vi "Fiducial Scan.vi"(8 "error in":errorcluster, 10 "input cluster":T1, 11 "Gantry In":refnum<k24>) -> (0 "error out":errorcluster, 1 "Not Found?":bool, 2 "output cluster":T1, 3 "Gantry Out":refnum<k24>)   [LabVIEW 2021, in "Component Tray.lvclass"]
uses:
  Component Tray.lvclass
  Find Component.ctl
  Controller/Camera/Machine Vision.ctl
  C:/Program Files (x86)/Aerotech/A3200/LabVIEW/2010/Bin/Aerotech.A3200.dll
  Program Files (x86)/Aerotech/A3200/LabVIEW/2010/Bin/Aerotech.A3200.dll
  Controller/Motion/A3200/A3200.lvclass
  Controller/Camera/Camera.lvclass
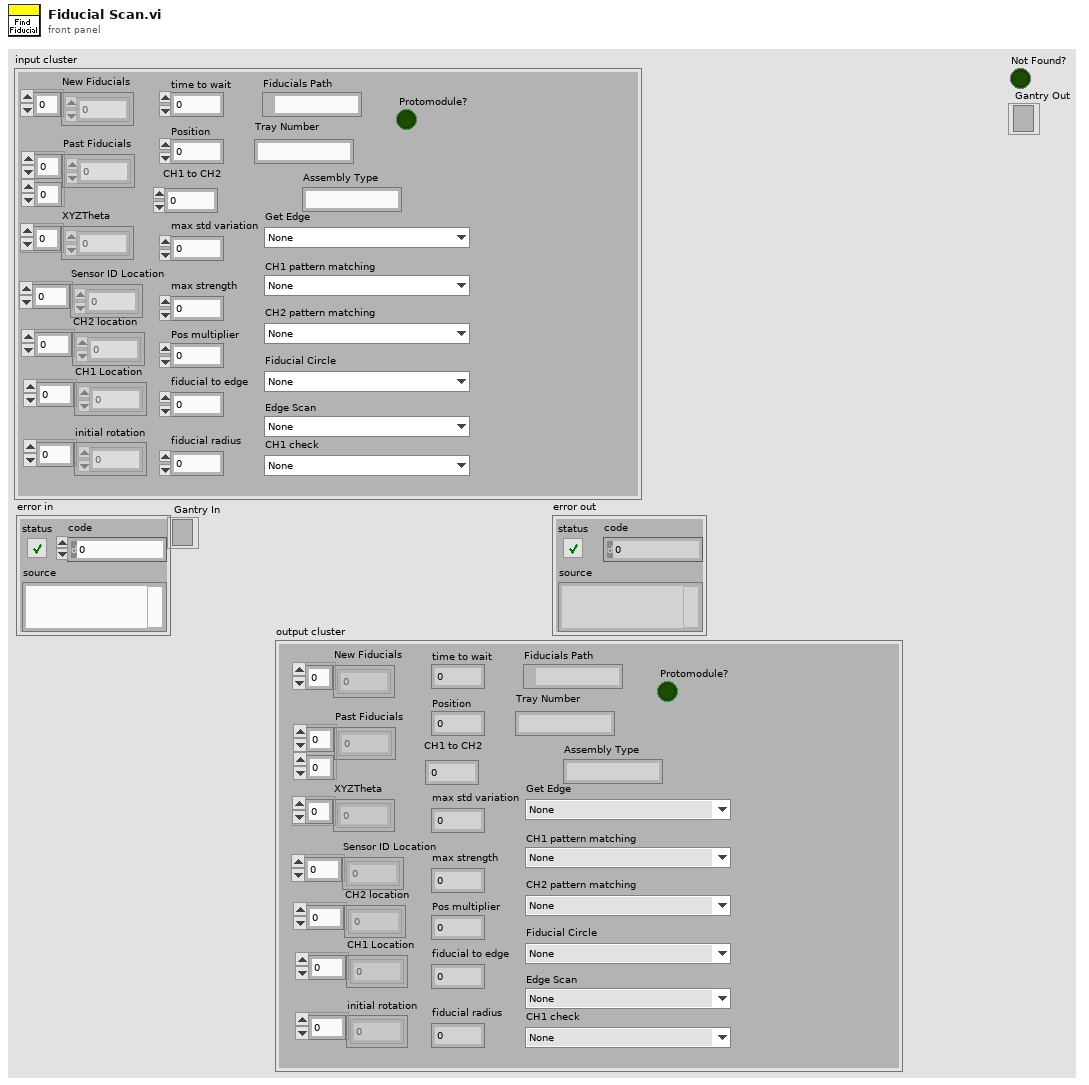
[diagram p1: front panel]
types:
  T1 = typedef "Component Tray.lvclass/Find Component.ctl" = cluster{"New Fiducials":dbl[], "Past Fiducials":dbl[][], "XYZTheta":dbl[], "Fiducials Path":path, "Position":i32, "CH1 Location":dbl[], "Sensor ID Location":dbl[], "initial rotation":dbl[], "CH2 location":dbl[], "max std variation":dbl, "max strength":dbl, "CH2 pattern matching":T2, "Fiducial Circle":T2, "Get Edge":T2, "Pos multiplier":dbl, "time to wait":u32, "fiducial to edge":dbl, "Protomodule?":bool, "Assembly Type":string, "CH1 to CH2":dbl, "Tray Number":string, "fiducial radius":dbl, "4 fiducials?":bool, "CH1 check":T2, "Edge Scan":T2, "CH1 pattern matching":T2, "Sensor Thickness":dbl}
  T2 = typedef "Camera.lvclass/Machine Vision.ctl" = enum16{"None", "Assembly Tray Circle", "Assembly Tray Fiducial", "Partial Hexaboard", "sensor edge init", "HB edge init", "sensor edge pos1", "sensor edge pos2", "HB edge pos1", "HB edge pos2", "Sensor CH1-2", "HB CH1", "HB CH2", "V3 Sensor Circle", "Hexaboard Circle", "sensor CH1 check", "HB CH1 check "}
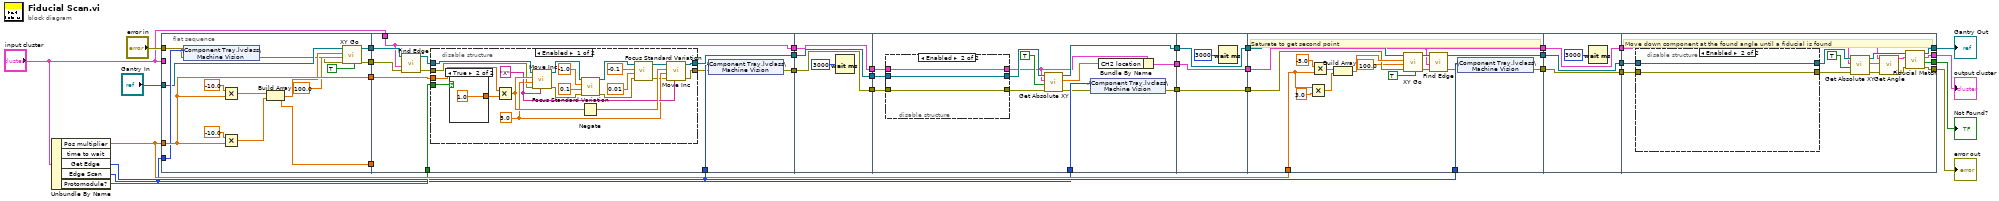
[diagram p0: block diagram]
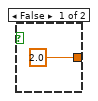
[diagram p2: hidden frame]
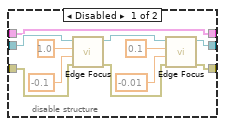
[diagram p4: hidden frame]
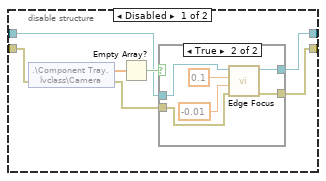
[diagram p5: hidden frame]
diagram:
  n1 = Unbundle By Name("input cluster") -> ("Pos multiplier"=w33:dbl, "Get Edge"=w2:T2, "Edge Scan"=w1:T2, "Protomodule?"=w6:bool)  [unwired: 1 out]
  n2 = flat-sequence {
    tunnel: w1 -> [w46]
    tunnel: w33 -> [w47]
    tunnel: "Gantry In" -> [w45]
    tunnel: [w34] -> w15
    tunnel: [w47] -> w14
    tunnel: [w35] -> w13
    tunnel: "error in" -> [w37]
    tunnel: [w38] -> w11
    tunnel: "input cluster" -> [_]
    tunnel: [w58] -> w5
    tunnel: [w55] -> w4
    tunnel: [w49] -> w3
    tunnel: w2 -> [w57]
    tunnel: w15 -> [w50]
    tunnel: w14 -> [w51]
    tunnel: w13 -> [w52]
    tunnel: w11 -> [_]
    tunnel: "input cluster" -> [w49]
    tunnel: w6 -> [w48]
    tunnel: w5 -> [w87]
    tunnel: [w87] -> w9
    tunnel: w4 -> [w86]
    tunnel: [w86] -> w8
    tunnel: [w84] -> w7
    tunnel: w3 -> [w84]
    tunnel: [w100] -> w21
    tunnel: [w96] -> w19
    tunnel: [w99] -> w17
    tunnel: w1 -> [w98]
    tunnel: w9 -> [w92]
    tunnel: w8 -> [w91]
    tunnel: w7 -> [w90]
    tunnel: w21 -> [w118]
    tunnel: [w118] -> w20
    tunnel: w19 -> [w117]
    tunnel: [w117] -> w18
    tunnel: w17 -> [w116]
    tunnel: [w116] -> w16
    tunnel: [w132] -> w27
    tunnel: [w135] -> w25
    tunnel: w2 -> [w134]
    tunnel: [w119] -> w23
    tunnel: w16 -> [w119]
    tunnel: w33 -> [w121]
    tunnel: w18 -> [w125]
    tunnel: w20 -> [w123]
    tunnel: w27 -> [w139]
    tunnel: [w139] -> w26
    tunnel: w25 -> [w138]
    tunnel: [w138] -> w24
    tunnel: w23 -> [w137]
    tunnel: [w137] -> w22
    tunnel: [w153] -> w32
    tunnel: [w152] -> w31
    tunnel: [w149] -> w29
    tunnel: [w148] -> w28
    tunnel: w22 -> [w141]
    tunnel: w24 -> [w145]
    tunnel: w26 -> [w143]
    frame #0 {
      n3 = shared-variable ".\\Component Tray.lvclass\\Machine Vision"(w46, error in=w37) -> (error out=w36:errorcluster)
      n4 = Multiply(x=-10.0, y=w47) -> (x*y=w42:dbl)
      n5 = Multiply(x=-10.0, y=w47) -> (x*y=w43:dbl)
      n6 = Build Array(w42, w43) -> (w38:dbl[])
      n7 = call "XY Go.vi"("Increment?"=TRUE, "error in (no error)"=w36, "Speed"=100.0, "XY In"=w38, "Gantry In"=w45) -> ("error out"=w34:errorcluster, "Gantry Out"=w35:refnum<k24>)  [unwired: 4 in, 1 out]
    }
    frame #1 {
      n8 = call "Find Edge.vi"("error in"=w50, "input cluster"=w49, "Gantry In"=w52) -> ("error out"=w53:errorcluster, "Gantry Out"=w54:refnum<k24>)  [unwired: 7 in]
      n9 = disable-structure shown="Enabled" {
        disable-tunnel: w54 -> [w77 w83]
        disable-tunnel: [w74 w83] -> w58
        disable-tunnel: [w69 w82] -> w56
        disable-tunnel: w53 -> [w60 w82]
        disable-tunnel: w51 -> [w79 _]
        disable-tunnel: w48 -> [w59 _]
        frame Enabled {
          w71 = "X" ("Axis")
          w70 = 5.0 ("Speed")
          n10 = case shown="True" w59 {
            tunnel: [2.0 ("y") 1.0 ("y")] -> w78
            frame False {
            }
            frame True {
            }
          }
          n11 = Multiply(x=w79, y=w78) -> (x*y=w73:dbl)
          n12 = call "Move Inc.vi"("Axis"=w71, "error in (no error)"=w60, "Speed"=w70, "Distance"=w73, "Gantry In"=w77) -> ("error out"=w75:errorcluster, "Gantry Out"=w76:refnum<k24>)  [unwired: 5 in]
          n13 = Negate(x=w73) -> (-x=w72:dbl)
          n14 = call "Focus Standard Variation.vi"("error in"=w75, "Scan Inc"=0.1, "Start Inc"=-1.0, "Gantry In"=w76) -> ("error out"=w68:errorcluster, "Gantry Out"=w66:refnum<k24>)  [unwired: 5 in, 1 out]
          n15 = call "Focus Standard Variation.vi"("error in"=w68, "Scan Inc"=0.01, "Start Inc"=-0.1, "Gantry In"=w66) -> ("error out"=w67:errorcluster, "Gantry Out"=w65:refnum<k24>)  [unwired: 5 in, 1 out]
          n16 = call "Move Inc.vi"("Axis"=w71, "error in (no error)"=w67, "Speed"=w70, "Distance"=w72, "Gantry In"=w65) -> ("error out"=w69:errorcluster, "Gantry Out"=w74:refnum<k24>)  [unwired: 5 in]
        }
        frame Disabled {
        }
      }
      n17 = shared-variable ".\\Component Tray.lvclass\\Machine Vision"(w57, error in=w56) -> (error out=w55:errorcluster)
    }
    frame #2 {
      n18 = Wait (ms)(milliseconds to wait=u32 3000) -> ()  [unwired: 1 out]
    }
    frame #3 {
      n19 = disable-structure shown="Enabled" {
        disable-tunnel: w92 -> [w111 w114]
        disable-tunnel: [w105 w114] -> w93
        disable-tunnel: [w104 w113] -> w94
        disable-tunnel: w91 -> [w110 w113]
        disable-tunnel: w90 -> [w109 w112]
        disable-tunnel: [w109 w112] -> w88
        frame Disabled {
          n20 = call "Edge Focus.vi"("error in"=w110, "Increment Size"=-0.1, "Position In"=1.0, "Gantry In"=w111) -> ("error out"=w103:errorcluster, "Gantry Out"=w106:refnum<k24>)  [unwired: 6 in]
          n21 = call "Edge Focus.vi"("error in"=w103, "Increment Size"=-0.01, "Position In"=0.1, "Gantry In"=w106) -> ("error out"=w104:errorcluster, "Gantry Out"=w105:refnum<k24>)  [unwired: 6 in]
        }
        frame Enabled {
        }
      }
      n22 = call "Get Absolute XY.vi"("error in (no error)"=w94, "Edge?"=TRUE, "input cluster"=w88, "Gantry In"=w93) -> ("error out"=w97:errorcluster, "Abs XY"=w95:dbl[], "Gantry Out"=w100:refnum<k24>)  [unwired: 5 in]
      n23 = shared-variable ".\\Component Tray.lvclass\\Machine Vision"(w98, error in=w97) -> (error out=w96:errorcluster)
      n24 = Bundle By Name(cluster=w88, "CH2 location"=w95) -> (w99:T1)
    }
    frame #4 {
      n25 = Wait (ms)(milliseconds to wait=u32 3000) -> ()  [unwired: 1 out]
    }
    frame #5 {
      # "Saturate to get second point"
      n26 = Multiply(x=w121, y=3.0) -> (x*y=w122:dbl)
      n27 = Multiply(x=-5.0, y=w121) -> (x*y=w128:dbl)
      n28 = Build Array(w128, w122) -> (w129:dbl[])
      n29 = call "XY Go.vi"("Increment?"=TRUE, "error in (no error)"=w125, "Speed"=100.0, "XY In"=w129, "Gantry In"=w123) -> ("error out"=w131:errorcluster, "Gantry Out"=w130:refnum<k24>)  [unwired: 4 in, 1 out]
      n30 = call "Find Edge.vi"("error in"=w131, "input cluster"=w119, "Gantry In"=w130) -> ("error out"=w133:errorcluster, "Gantry Out"=w135:refnum<k24>)  [unwired: 7 in]
      n31 = shared-variable ".\\Component Tray.lvclass\\Machine Vision"(w134, error in=w133) -> (error out=w132:errorcluster)
    }
    frame #6 {
      n32 = Wait (ms)(milliseconds to wait=u32 3000) -> ()  [unwired: 1 out]
    }
    frame #7 {
      # "Move down component at the found angle until a fiducial is found"
      n33 = disable-structure shown="Enabled" {
        disable-tunnel: w145 -> [w157 w171]
        disable-tunnel: [w155 w171] -> w144
        disable-tunnel: w143 -> [w161 w170]
        disable-tunnel: [w156 w170] -> w142
        frame Disabled {
          n34 = shared-variable ".\\Component Tray.lvclass\\Camera"(error in=w161) -> (w160:dbl[], error out=w158:errorcluster)
          n35 = Empty Array?(array=w160) -> (empty?=w159:bool)
          n36 = case shown="True" w159 {
            tunnel: w158 -> [w162 w169]
            tunnel: w157 -> [w163 w168]
            tunnel: [w162 w167] -> w156
            tunnel: [w163 w166] -> w155
            frame False {
            }
            frame True {
              n37 = call "Edge Focus.vi"("error in"=w169, "Increment Size"=-0.01, "Position In"=0.1, "Gantry In"=w168) -> ("error out"=w167:errorcluster, "Gantry Out"=w166:refnum<k24>)  [unwired: 6 in]
            }
          }
        }
        frame Enabled {
        }
      }
      n38 = call "Get Absolute XY.vi"("error in (no error)"=w142, "Edge?"=TRUE, "input cluster"=w141, "Gantry In"=w144) -> ("error out"=w146:errorcluster, "Abs XY"=w147:dbl[], "Gantry Out"=w154:refnum<k24>)  [unwired: 5 in]
      n39 = call "Get Angle.vi"("error in"=w146, "array"=w147, "input cluster"=w141) -> ("error out"=w151:errorcluster, "output cluster"=w150:T1)  [unwired: 7 in]
      n40 = call "Fiducial Match.vi"("error in (no error)"=w151, "input cluster"=w150, "Gantry In"=w154) -> ("error out"=w152:errorcluster, "Not Found?"=w149:bool, "output cluster"=w148:T1, "Gantry Out"=w153:refnum<k24>)  [unwired: 5 in]
    }
  }
  "Not Found?" <- w29
  "error out" <- w31
  "Gantry Out" <- w32
  "output cluster" <- w28
